vi "MCLScanAll.vi"() -> ()   [LabVIEW 2013]
uses:
  <vilib>/Analysis/NI_AALBase.lvlib
  <vilib>/Analysis/baseanly.llb/Mean (DBL).vi
  <vilib>/vision/NI_Vision_Development_Module.lvlib
  <vilib>/vision/Image Controls.llb/IMAQ Image.ctl
panel:
  in  "MCLScanning":bool
  in  "In Images":T2
  in  "APD 2 Cts":dbl[](array[numeric])
  in  "Trap Raw":waveform(dbl)[](array[waveform])
  in  "APD 1 Cts":dbl[](array[numeric])
  in  "Scan steps (MCL)":u64=40 caption="Scan steps (x)"
  in  "N APD Samp/step":dbl=3.0
  in  "Scan lines (y)":u64=20
  out "Cycles/step (MCL)":u64=2000 caption="Cycles/step" format="%.0p"
  out "Data map":dbl[][](graph)=[[-0.01671932143166878, -0.016392818706373227, -0.016060241502617766, -0.016885058281480972, -0.016633639866051188, -0.01614297111485056, -0.01624632439809061, -0.016223291898502697, -0.016322135358181895, -0.015998827366942206, -0.01674383457317074, -0.016349622303473588, -0.01611571290004051, -0.015972334649942688, -0.016306900004507047, -0.016265804263496074, -0.0160006281874421, -0.01579815848604542, -0.015557994770877373, -0.01623934207097493], [-0.016401746716030643, -0.016486228679580477, -0.016405819418185925, -0.017006941359896506, -0.01609698301441303, -0.0159938373980257, -0.015449969664593804, -0.016068061784641922, -0.016115383931390913, -0.015648222289449794, -0.01653040435156989, -0.01664368093936457, -0.015976629115606142, -0.015769041987412753, -0.015716784490458328, -0.016104708313091028, -0.015807740113897233, -0.016007795937736217, -0.015716865824611653, -0.016131560547170874], [-0.016881180243279052, -0.016682362901092443, -0.01653521208533211, -0.016569663649832547, -0.016584350108926265, -0.015788034358096, -0.01572997381191265, -0.016848256863673278, -0.016450971094654886, -0.016646544202256155, -0.016533647976865372, -0.01643411945121718, -0.01642968729491641, -0.015287525792493872, -0.015664412933211656, -0.016705160893495323, -0.01634751515697455, -0.016385950364931786, -0.01641611962972788, -0.016336369365154098], [-0.016944386833653874, -0.017209095062396696, -0.01643647162326984, -0.0169434622427136, -0.01645749558522405, -0.016283892481898044, -0.016603972603686925, -0.016019804038190342, -0.01633990863890397, -0.016779562572954584, -0.01649257003377154, -0.01633196294664365, -0.01681717360495772, -0.016151141680784836, -0.015631110690343758, -0.01616762209708058, -0.01570812545409377, -0.016238042109499973, -0.016140009377557954, -0.015480352129179791], [-0.016627380272623872, -0.016987040432100503, -0.0162998105424607, -0.01635693474229572, -0.016728613514399027, -0.015877063835195653, -0.01632422175035657, -0.015987062444069455, -0.016082210905250194, -0.016795453503208664, -0.0170165982501747, -0.016041147401410074, -0.015844635002206515, -0.01588368721722097, -0.016415515701510675, -0.01625686223052733, -0.015522307984761095, -0.016125254990784654, -0.016133227363549094, -0.016093654313254407], [-0.016918226627058684, -0.016546339201955095, -0.016238630263811032, -0.01698719582491472, -0.016111760237599002, -0.016169388046078873, -0.01635628471807927, -0.016477982760217016, -0.016022494806163096, -0.01635452184408291, -0.016437829589091835, -0.01620151587720066, -0.016192846971583803, -0.016361330735626047, -0.015920360440429684, -0.015596058601637491, -0.015839057608204695, -0.01590683226225114, -0.016147455226815495, -0.016061133185195295], [-0.016634948322751798, -0.016569012123295146, -0.01662465918442623, -0.01677966319575081, -0.016244237674368125, -0.016934028324529424, -0.015994902143504568, -0.01577806108898649, -0.015702882269567658, -0.01637426003303808, -0.016516796952512437, -0.01646180977161214, -0.017050841082784957, -0.015210920961454804, -0.016180578875882937, -0.01607665952058283, -0.01643056573904152, -0.01624726697921726, -0.016811320756287537, -0.015704237088347145], [-0.016797771368752906, -0.01616083928333069, -0.016453251971550422, -0.01638112181272177, -0.01590261356594244, -0.01608147749759244, -0.016020370516697566, -0.01666407664114518, -0.01638481284701757, -0.016175328500489604, -0.015634096607040564, -0.01659680945708638, -0.01626086024191585, -0.016096523812787963, -0.015760521307245458, -0.01615157630765101, -0.01563169067138887, -0.016252628883934674, -0.016238504839935688, -0.016296984466382107], [-0.01667963634531472, -0.015869270181190567, -0.01639782773103042, -0.01636439382881424, -0.01666285543553242, -0.016692875783958446, -0.016121724588237546, -0.016079967645743654, -0.01632967716613466, -0.0165840590606689, -0.01625421166976198, -0.016098422085292646, -0.016839026057991122, -0.01618499247497865, -0.015391600029151147, -0.016339655626827314, -0.015612166346566772, -0.015935379715422582, -0.015751812989013417, -0.016043659821299468], [-0.016548348623009697, -0.016991017407413864, -0.016507403110123067, -0.016536793878207376, -0.016691120016137963, -0.01577327808799238, -0.016241167864690632, -0.016068735698142586, -0.015840387814149363, -0.016134357225980472, -0.015841333026290365, -0.0163038114660657, -0.01664004009343323, -0.015517995684912076, -0.01510255011893393, -0.016011490555515644, -0.01579492187645071, -0.016061693314939115, -0.016070791499276448, -0.015958266458419586], [-0.017158052821315092, -0.016990745992594425, -0.01659770916824297, -0.016038631482428484, -0.016146804022232154, -0.01576224906436341, -0.016188682344964726, -0.016682643876198163, -0.016363274145684666, -0.01639850086318443, -0.015896821220835786, -0.015725853678146523, -0.01601090474694708, -0.015561700057052, -0.015999978841264924, -0.01601836056022779, -0.016765653382201824, -0.016096916088969352, -0.016073837821775124, -0.015692878955540758], [-0.01663419671959083, -0.016709422884628247, -0.017440867448447667, -0.016794212435564802, -0.016747490720603195, -0.017381751349696366, -0.016447004176656708, -0.016200072448833015, -0.016045160782039845, -0.01632124390318996, -0.01679169430451878, -0.016160654157203025, -0.016749084172300182, -0.015317451826774697, -0.01616958983467165, -0.015522373654827837, -0.016042029406509332, -0.016273918604509642, -0.016417636335760946, -0.01644358854973573], [-0.016334373306253872, -0.016757773312361682, -0.016379901767213538, -0.016648254461466998, -0.016415141976627915, -0.016163802224577726, -0.01585938187523836, -0.01585373106879133, -0.015975877635193418, -0.01599748687305492, -0.016737850820893803, -0.01594503246026053, -0.01605934628998727, -0.0158171814426758, -0.015143820145612868, -0.016535815039113604, -0.01611350163485256, -0.01603586147994221, -0.016191023597649318, -0.015673182413705102], [-0.016700857633048308, -0.017051706885756718, -0.016395162126784154, -0.016864165985049667, -0.01667278712452, -0.016023236569300325, -0.015936447644162688, -0.01626053315184134, -0.016666644977778797, -0.01651990276982608, -0.01690611112853018, -0.016570014742366936, -0.016014494913507715, -0.016334286074074115, -0.01621235686701924, -0.01653022812336152, -0.01583634924223019, -0.016281303974484927, -0.01653990312391212, -0.015384206653677268], [-0.016471441301573585, -0.01647096314202187, -0.016715886966535524, -0.015878302888681167, -0.016818970876684446, -0.016713152489800882, -0.0154648252478201, -0.016328530500277577, -0.015836781582585016, -0.01591923201699931, -0.016315094505816256, -0.015951841421804724, -0.01608430179945204, -0.015957272458344565, -0.015751249520465478, -0.016350306857141315, -0.015517909552404317, -0.015884662571158274, -0.016211720964471307, -0.01537858018482844], [-0.01674440523726064, -0.016870567772511377, -0.016213148874409115, -0.016888734754126403, -0.017090609693170035, -0.01659256562080198, -0.01625635717081822, -0.016107107745803876, -0.016234190134722645, -0.016577197956586683, -0.01658670958631228, -0.016563728816596346, -0.016688515093891267, -0.016736196160361996, -0.015994597797780702, -0.016061666241292242, -0.015206770358209283, -0.01656914278587982, -0.01606315534154764, -0.015681866815853374], [-0.016944331036564515, -0.017205260427342613, -0.01677120483170293, -0.016402843466637763, -0.01674116281665193, -0.016423395631415146, -0.01525500299962603, -0.01627542397053335, -0.016664853908603776, -0.01620332976021642, -0.015950564835878013, -0.01610107356411497, -0.016396683154864377, -0.015976631236977498, -0.015478300298060717, -0.015835627632208554, -0.01604600189786053, -0.015850180758366084, -0.01603596051783181, -0.015769623989901102], [-0.016857923835780924, -0.016573198672727902, -0.016660307411618773, -0.016198760579099178, -0.016151481374992453, -0.01623511193332007, -0.015818969815924802, -0.01644510963983431, -0.015972042272190907, -0.01666642359581892, -0.01666443700190194, -0.016438254918363447, -0.016138118663893655, -0.015691974269895034, -0.016587077315345165, -0.015965118060360686, -0.015699839910512218, -0.01561194620613338, -0.016186792034230305, -0.016197922335520733], [-0.016756662992071368, -0.017021980605505502, -0.01671540550240299, -0.016161860765568574, -0.016256637402529132, -0.01604906368842445, -0.016092507257301394, -0.01617438393323743, -0.016105543848009572, -0.016246592326198385, -0.016142744624025374, -0.016159689527728567, -0.016177575339496836, -0.015961391152738445, -0.015789242903564853, -0.016290502978789936, -0.01590902706214275, -0.016035878036151207, -0.0163699057102928, -0.016166856731619543], [-0.016230743921604517, -0.01699457586491366, -0.01691575006710251, -0.01691567874763252, -0.016632348348462205, -0.01564006866069024, -0.015669555325846102, -0.01675726036853814, -0.015659388136628594, -0.01633203630678029, -0.016275904140963263, -0.01599466989252362, -0.01670183436780044, -0.016544315654085533, -0.015882735536646285, -0.01634814491721433, -0.015693511174422668, -0.015857069610244905, -0.015293298228102974, -0.01570879180052374], [-0.016746550537387085, -0.016635756849929545, -0.01704192789682773, -0.01592942336549498, -0.016565335498658518, -0.016559981627150607, -0.016370390094235444, -0.016204117687222342, -0.01636993721064581, -0.016019023809705737, -0.01624713908528634, -0.01653713290533686, -0.01654191191022731, -0.015871787270804183, -0.016600435605206076, -0.016053794928515903, -0.015786397557799592, -0.016167422435048453, -0.016149009764007245, -0.015779827376486453], [-0.017141787830569893, -0.01685604196926299, -0.016770676218784503, -0.01657265724540346, -0.016973351148096293, -0.016347677914333066, -0.015700463473615457, -0.0157292679709582, -0.016282549721629708, -0.015799962485816943, -0.0169651499113691, -0.017005390716294616, -0.01616841590634147, -0.01579805772887789, -0.015884669429112312, -0.01687947774540062, -0.015546104827296667, -0.01606408203496036, -0.015764690031214893, -0.016077969368821936], [-0.01755128513645066, -0.016614441354853425, -0.01642295621649906, -0.016572002735089818, -0.016539344978417192, -0.01665672671509038, -0.01610564101766388, -0.0167710479608722, -0.01604147346071364, -0.015915051759660022, -0.01690954942974296, -0.01618215110656205, -0.01687103577661275, -0.015704550539293104, -0.01567934362211993, -0.015968805810754147, -0.01586985536309292, -0.015848872001954256, -0.015923479964089694, -0.015604572794266433], [-0.01700702905775247, -0.016405242404623068, -0.016957584669743626, -0.01649808356316003, -0.015831866505709048, -0.01650461850371917, -0.015987113078007254, -0.015834023912635466, -0.015505062044615166, -0.016233666617861173, -0.016028249584376462, -0.016292798595496677, -0.016811560188299345, -0.015802581883183398, -0.015195148613460024, -0.015765465657774175, -0.016294889918615045, -0.01647530657977607, -0.016354233471026363, -0.01618598563271133], [-0.016283357847285636, -0.01655641981831666, -0.016127059444156554, -0.016293855360523378, -0.01631947219897442, -0.016398508430939616, -0.0164960599809452, -0.01635229032278839, -0.016150072161158744, -0.01646190473964058, -0.016283962555137702, -0.01689040784367708, -0.016767163139998632, -0.016438000493173108, -0.015954956500429416, -0.016569056147695202, -0.016605504963760735, -0.015329313107534112, -0.01578842030659742, -0.015421959499234628], [-0.016479987599589248, -0.01644678482494596, -0.016512996052180717, -0.01623094473834884, -0.016604746810030113, -0.016230213519226107, -0.016359208382350467, -0.01609761921903255, -0.016464485575532387, -0.015985272322973462, -0.015774520381458212, -0.01632178510310122, -0.016823351362691343, -0.01643553466150876, -0.015434648968053383, -0.01640702032901096, -0.015639626970513753, -0.01608966370811705, -0.016018362361111357, -0.01607982188546427], [-0.016959739645157706, -0.016680901866661726, -0.015836205448559966, -0.016650560318028734, -0.015979362423611275, -0.015641297610719303, -0.015788746501915876, -0.016033508703118756, -0.01595573902096323, -0.016363948579213562, -0.016349864006002027, -0.016495398899173445, -0.016242648234899834, -0.016920033344786076, -0.016276181128461735, -0.016473741446416813, -0.015963577017676644, -0.015565621002678179, -0.01634988477510272, -0.016759987490697584], [-0.016465195958807775, -0.016666490625723715, -0.016658908615375, -0.01597417902764041, -0.016394946754303752, -0.016153528909152313, -0.016275277887248356, -0.016575820504070977, -0.016165440248126276, -0.0158334592734765, -0.016393067206609387, -0.016885479811953534, -0.016471593134372298, -0.017124297138208497, -0.01548599428740715, -0.016309544928836586, -0.015739577267293366, -0.016315386973421362, -0.016361118135948566, -0.016635949477566882], [-0.016680470580762462, -0.016967020008211, -0.017070403001069857, -0.015793158201855152, -0.01661718510493328, -0.01621301409151063, -0.015497330917384148, -0.016267684516616924, -0.015545683307124036, -0.01584462817622427, -0.016830529260392843, -0.016203294725707643, -0.016943290418910587, -0.015581438668509352, -0.015578492450734066, -0.01643368853494311, -0.016285119780950222, -0.015912568651561352, -0.015719368411857025, -0.015732642681635923], [-0.017056323385982973, -0.017071971641855074, -0.01624203196673346, -0.016577086084052214, -0.016198385464505236, -0.015959998936922397, -0.015388246890736087, -0.01690871560472578, -0.016520770777269024, -0.016719342780151844, -0.01589885976225658, -0.016316317143634285, -0.015927259253864068, -0.01613903479860508, -0.015938319643326725, -0.015996730877187566, -0.01552190097834432, -0.016279927776335308, -0.015995176436170485, -0.015804091652970826], [-0.017190435316337342, -0.016575163169333516, -0.01629659819256952, -0.016774256975583077, -0.015978440181354282, -0.016162892801179076, -0.01620143768882657, -0.016215940324925678, -0.016085616640623322, -0.01624795446292185, -0.015590279490139558, -0.016351775677783426, -0.01628162630120476, -0.016736583715483217, -0.015290607493835316, -0.01675006130238602, -0.016112399997689694, -0.016085396155956493, -0.01584495781031281, -0.016031709625742012], [-0.017226310157841672, -0.0164663033859778, -0.01638852606295136, -0.01642215259901681, -0.016566243818266997, -0.016484045986143257, -0.016452209817223822, -0.016464707609223313, -0.01598467645947642, -0.016476401570535384, -0.015529223129381136, -0.016802343788985992, -0.016417294815804, -0.016305476633183012, -0.015407470515554668, -0.01588918182788552, -0.015839354895906106, -0.016859219988342257, -0.016188952756112908, -0.015382351679335257], [-0.017044276140355946, -0.016525294382434108, -0.01600036800318285, -0.01692841042125611, -0.016063543400203904, -0.0167008216867912, -0.01583944304325613, -0.015982843969462788, -0.01610446772754332, -0.01650934416727942, -0.016660683575282727, -0.016326108469991264, -0.01614299940648814, -0.016050548764700443, -0.016131072933532012, -0.016315196635999143, -0.016225473554238007, -0.01551847935196565, -0.015874550726858914, -0.01566897000262655], [-0.016174756903461544, -0.01692999553661901, -0.01705167048362926, -0.01660949009366751, -0.016107419352032235, -0.016188509519945497, -0.015585853922651487, -0.01612262091090234, -0.016426426055949322, -0.01609822137272688, -0.016735004284984756, -0.016043599908818165, -0.016651804571551146, -0.01556136051538674, -0.015408827232157843, -0.015855874683892428, -0.015887023972496795, -0.01599811437353065, -0.015655637769778918, -0.015893480415302176], [-0.016396467105890343, -0.01690556505247584, -0.0163054855200399, -0.016446662941364928, -0.01622691165873451, -0.016690239637868323, -0.015785441074554568, -0.016620593981308673, -0.015765446409343138, -0.016270811628848948, -0.016094841434208293, -0.01632812303243944, -0.01619217328151394, -0.015836234359203484, -0.016074598803568225, -0.01532030760600064, -0.01657169575010852, -0.016393493124135967, -0.01597552762388542, -0.015565046037824628], [-0.016299520764774443, -0.016637551393085426, -0.016299287907039765, -0.01610813956937386, -0.016305200311999217, -0.016601228593523636, -0.016288899767132464, -0.016305235511310533, -0.016063090550620947, -0.01683118193989227, -0.015518909238992087, -0.01620458965118359, -0.01645647074542291, -0.015677575909554008, -0.015332584749786342, -0.016079840062543812, -0.016278322310175185, -0.01605786016548567, -0.01657700147769983, -0.01606751816440997], [-0.016441387384698882, -0.017325914631361444, -0.017225293509456174, -0.016118796157285526, -0.016362377734664042, -0.01516634537172325, -0.01608508664570788, -0.01572299536201756, -0.01616493137153105, -0.01621315960010322, -0.016750280429064943, -0.016228195768808316, -0.01653543568323192, -0.01645026349483051, -0.016050647149129828, -0.01642593239180811, -0.0161192309302286, -0.01629438826737352, -0.015557310160813994, -0.016021567325025916], [-0.01686693458295582, -0.016740786564424494, -0.01648453245605215, -0.01640092243822592, -0.01555424864442638, -0.01667099748425638, -0.016069415470156286, -0.01638225749592203, -0.01607630099787768, -0.01614344420814296, -0.016216929728619375, -0.016309670684273796, -0.015741358140653132, -0.015770999475234804, -0.01601963602183988, -0.01615265943136728, -0.016152653946118384, -0.01698528285009184, -0.015969420465915152, -0.01578449323306024], [-0.01598619419452168, -0.016362732490235912, -0.016433844312774552, -0.016357999277320685, -0.015969441982301692, -0.01621147526376268, -0.016085473373391473, -0.016306341052304336, -0.015855664982231947, -0.015900633884010838, -0.016902356755211914, -0.016434765274207237, -0.016180164153866673, -0.015973977144992546, -0.01589274164800459, -0.01640268056199417, -0.016415161422386984, -0.01617112040367598, -0.016354725082739732, -0.016206639631885546], [-0.016048964224847716, -0.016745007333129024, -0.017180534108641177, -0.016329775174222558, -0.016582289070660373, -0.016075138720435006, -0.016345162602564738, -0.016090296577092385, -0.016153752753705675, -0.016379459268123033, -0.016228628993078524, -0.016712275509199688, -0.015795168051192618, -0.015386431874568587, -0.01610093851445945, -0.01633598707495066, -0.015921284689633122, -0.016330315102764423, -0.015994974665173196, -0.015537812293197398]]
  out "Waveform Graph":dbl[](graph)=[5.0, 4.0, 2.0, 2.0, 5.0, 3.0, 2.0, 4.0, 0.0, 5.0, 4.0, 3.0, 5.0, 2.0, 4.0, 1.0, 5.0, 3.0, 0.0, 2.0, 2.0, 4.0, 2.0, 1.0, 2.0, 8.0, 2.0, 4.0, 4.0, 3.0, 3.0, 1.0, 5.0, 5.0, 3.0, 2.0, 7.0, 2.0, 4.0, 4.0, 1.0, 1.0, 3.0, 4.0, 3.0, 9.0, 0.0, 6.0, 4.0, 5.0, 2.0, 4.0, 4.0, 4.0, 4.0, 2.0, 3.0, 6.0, 3.0, 4.0, 4.0, 5.0, 5.0, 8.0, 5.0, 4.0, 4.0, 7.0, 4.0, 3.0, 1.0, 4.0, 5.0, 4.0, 2.0, 3.0, 3.0, 1.0, 2.0, 1.0] caption="APD Line Scan"
  in  "Channel":i32=4
  out "Detection Laser X":T1(plugin-control)
  out "APD 1":T1(plugin-control) caption="APD 1 (Cy3)"
  out "Detection Laser Y":T1(plugin-control)
  out "APD 2":T1(plugin-control) caption="APD 2 (Cy5)"
types:
  T1 = typedef "IMAQ Image.ctl" = refnum<image>
  T2 = cluster{"New Image":T1, "New Image":T1, "New Image":T1, "New Image":T1}
  T3 = cluster{"Origin Pixel":cluster{"X":sgl, "Y":sgl}, "Angle Relative to Horizontal (deg)":sgl, "Axis Reference":u32}
  T4 = typedef "Simple Grid Descriptor" = cluster{"X Step":sgl, "Y Step":sgl, "Unit":T5}
  T5 = typedef "Image Unit" = enum32{"Undefined", "Angström", "Micrometer", "Millimeter", "Centimeter", "Meter", "Kilometer", "Microinch", "Inch", "Feet", "Nautical miles", "Standard miles", "Steps"}
diagram:
  w18 = u32 0 items=["Horizontal", "Vertical", "Central", "1st Diagonal", "2nd Diagonal"] ("Type of Symmetry")
  w44 = u32 0 items=["Horizontal", "Vertical", "Central", "1st Diagonal", "2nd Diagonal"] ("Type of Symmetry")
  w47 = u32 0 items=["Horizontal", "Vertical", "Central", "1st Diagonal", "2nd Diagonal"] ("Type of Symmetry")
  w76 = u32 0 items=["Horizontal", "Vertical", "Central", "1st Diagonal", "2nd Diagonal"] ("Type of Symmetry")
  n1 = local read "Scan lines (y)"() -> (w7:u64)
  n2 = local read "Cycles/step (MCL)"() -> (w61:u64)
  n3 = Index Array(array="Trap Raw", index=10) -> (element=w110:waveform(dbl))
  n4 = Index Array(array="Trap Raw", index=11) -> (element=w107:waveform(dbl))
  n5 = Index Array(array="Trap Raw", index="Channel") -> (element=w106:waveform(dbl))
  n6 = Unbundle("In Images") -> ("New Image"=w11:T1, "New Image"=w10:T1, "New Image"=w9:T1, "New Image"=w8:T1)
  n7 = Unbundle By Name(w110) -> ("Y"=w63:dbl[])
  n8 = Unbundle By Name(w107) -> ("Y"=w65:dbl[])
  n9 = Unbundle By Name(w106) -> ("Y"=w70:dbl[])
  n10 = call "downsample 1D array - double.vi"("Ave N"=w61, "Array In"=w63) -> ("Array Out"=w62:dbl[])  [unwired: 1 out]
  n11 = call "downsample 1D array - double.vi"("Ave N"=w61, "Array In"=w65) -> ("Array Out"=w64:dbl[])  [unwired: 1 out]
  n12 = call "downsample 1D array - double.vi"("Ave N"=w61, "Array In"=w70) -> ("Array Out"=w69:dbl[])  [unwired: 1 out]
  n13 = local read "Scan steps (MCL)"() -> (w20:u64)
  n14 = local read "N APD Samp/step"() -> (w22:dbl)
  n15 = feedback #1("APD 1 Cts") -> (w130:dbl[])
  n16 = Build Array (concatenate)(w130, "APD 1 Cts") -> (w112:dbl[])
  n17 = feedback #2("APD 2 Cts") -> (w38:dbl[])
  n18 = Build Array (concatenate)(w38, "APD 2 Cts") -> (w37:dbl[])
  n19 = Select(t="APD 1 Cts", s="MCLScanning", f=w112) -> (s? t:f=w116:dbl[])
  n20 = feedback-in #1(w116) -> ()
  n21 = Select(t="APD 2 Cts", s="MCLScanning", f=w37) -> (s? t:f=w21:dbl[])
  n22 = feedback-in #2(w21) -> ()
  n23 = feedback #3(w62) -> (w118:dbl[])
  n24 = Build Array (concatenate)(w118, w62) -> (w109:dbl[])
  n25 = feedback #4(w69) -> (w128:dbl[])
  n26 = Build Array (concatenate)(w128, w69) -> (w127:dbl[])
  n27 = feedback #5(w64) -> (w120:dbl[])
  n28 = Build Array (concatenate)(w120, w64) -> (w121:dbl[])
  n29 = Select(t=w64, s="MCLScanning", f=w121) -> (s? t:f=w67:dbl[])
  n30 = feedback-in #5(w67) -> ()
  n31 = Select(t=w62, s="MCLScanning", f=w109) -> (s? t:f=w66:dbl[])
  n32 = feedback-in #3(w66) -> ()
  n33 = Select(t=w69, s="MCLScanning", f=w127) -> (s? t:f=w68:dbl[])
  n34 = feedback-in #4(w68) -> ()
  n35 = Multiply(x=w20, y=u64 2) -> (x*y=w6:u64)
  n36 = call "integrate 1D array interval - double.vi"("Ave N"=w22, "Array In"=w21) -> ("Array Out"=w33:dbl[])  [unwired: 1 out]
  n37 = call "integrate 1D array interval - double.vi"("Ave N"=w22, "Array In"=w116) -> ("Array Out"=w115:dbl[])  [unwired: 1 out]
  n38 = Array Size(array=w33) -> (size(s)=w34:i32)
  n39 = Array Size(array=w115) -> (size(s)=w117:i32)
  n40 = Multiply(x=w7, y=w6) -> (x*y=w36:u64)
  n41 = Multiply(x=w7, y=w6) -> (x*y=w125:u64)
  n42 = call-poly <vilib>:"Mean.vi"("X"=w66) -> ("mean"=w50:dbl)  [unwired: 1 out]
  n43 = Subtract(x=w36, y=w34) -> (x-y=w27:u64)
  n44 = call-poly <vilib>:"Mean.vi"("X"=w68) -> ("mean"=w55:dbl)  [unwired: 1 out]
  n45 = call-poly <vilib>:"Mean.vi"("X"=w67) -> ("mean"=w53:dbl)  [unwired: 1 out]
  n46 = call-poly <vilib>:"Mean.vi"("X"=w33) -> ("mean"=w24:dbl)  [unwired: 1 out]
  n47 = Subtract(x=w125, y=w117) -> (x-y=w60:u64)
  n48 = call-poly <vilib>:"Mean.vi"("X"=w115) -> ("mean"=w57:dbl)  [unwired: 1 out]
  n49 = Initialize Array(1.0 ("element"), w27) -> (w23:dbl[])
  n50 = Initialize Array(1.0 ("element"), w60) -> (w51:dbl[])
  n51 = Multiply(x=w23, y=w24) -> (x*y=w25:dbl[])
  n52 = Multiply(x=w51, y=w53) -> (x*y=w54:dbl[])
  n53 = Multiply(x=w51, y=w55) -> (x*y=w56:dbl[])
  n54 = Multiply(x=w51, y=w50) -> (x*y=w52:dbl[])
  n55 = Multiply(x=w51, y=w57) -> (x*y=w58:dbl[])
  n56 = Build Array (concatenate)(w66, w52) -> (w119:dbl[])
  n57 = Build Array (concatenate)(w68, w56) -> (w123:dbl[])
  n58 = Build Array (concatenate)(w67, w54) -> (w122:dbl[])
  n59 = Build Array (concatenate)(w33, w25) -> (w35:dbl[])
  n60 = Build Array (concatenate)(w115, w58) -> (w124:dbl[])
  n61 = Reshape Array(w119, w7, w6) -> (w86:dbl[][])
  n62 = Reshape Array(w35, w7, w6) -> (w31:dbl[][])
  n63 = Reshape Array(w123, w7, w6) -> (w78:dbl[][])
  n64 = Reshape Array(w122, w7, w6) -> (w93:dbl[][])
  n65 = Reshape Array(w124, w7, w6) -> (w103:dbl[][])
  n66 = Array Subset(array=w93, index (col)=0 ("index"), length (col)=w20) -> (w98:dbl[][])  [unwired: 2 in]
  n67 = Array Subset(array=w93, index (col)=w20) -> (w96:dbl[][])  [unwired: 3 in]
  n68 = Array Subset(array=w78, index (col)=0 ("index"), length (col)=w20) -> (w84:dbl[][])  [unwired: 2 in]
  n69 = Array Subset(array=w78, index (col)=w20) -> (w82:dbl[][])  [unwired: 3 in]
  n70 = Array Subset(array=w31, index (col)=0 ("index"), length (col)=w20) -> (w30:dbl[][])  [unwired: 2 in]
  n71 = Array Subset(array=w31, index (col)=w20) -> (w28:dbl[][])  [unwired: 3 in]
  n72 = Array Subset(array=w103, index (col)=0 ("index"), length (col)=w20) -> (w102:dbl[][])  [unwired: 2 in]
  n73 = Array Subset(array=w103, index (col)=w20) -> (w100:dbl[][])  [unwired: 3 in]
  n74 = Array Subset(array=w86, index (col)=0 ("index"), length (col)=w20) -> (w91:dbl[][])  [unwired: 2 in]
  n75 = Array Subset(array=w86, index (col)=w20) -> (w89:dbl[][])  [unwired: 3 in]
  n76 = for {
    tunnel: w98 -> [w132] mode=indexing
    tunnel: [w131] -> w97 mode=indexing
    workers-P: _ -> [_]
    n77 = Reverse 1D Array(array=w132) -> (reversed array=w131:dbl[])
  }
  n78 = for {
    tunnel: w84 -> [w134] mode=indexing
    tunnel: [w133] -> w83 mode=indexing
    workers-P: _ -> [_]
    n79 = Reverse 1D Array(array=w134) -> (reversed array=w133:dbl[])
  }
  n80 = for {
    tunnel: w30 -> [w136] mode=indexing
    tunnel: [w135] -> w29 mode=indexing
    workers-P: _ -> [_]
    n81 = Reverse 1D Array(array=w136) -> (reversed array=w135:dbl[])
  }
  n82 = for {
    tunnel: w102 -> [w138] mode=indexing
    tunnel: [w137] -> w101 mode=indexing
    workers-P: _ -> [_]
    n83 = Reverse 1D Array(array=w138) -> (reversed array=w137:dbl[])
  }
  n84 = for {
    tunnel: w91 -> [w140] mode=indexing
    tunnel: [w139] -> w90 mode=indexing
    workers-P: _ -> [_]
    n85 = Reverse 1D Array(array=w140) -> (reversed array=w139:dbl[])
  }
  n86 = Index Array(array=w103, index (row)=0) -> (element=→"Waveform Graph":dbl[])  [unwired: 1 in]
  n87 = Add(x=w97, y=w96) -> (x+y=w95:dbl[][])
  n88 = Add(x=w83, y=w82) -> (x+y=w81:dbl[][])
  n89 = Add(x=w29, y=w28) -> (x+y=w13:dbl[][])
  n90 = Add(x=w101, y=w100) -> (x+y=w75:dbl[][])
  n91 = Add(x=w90, y=w89) -> (x+y=w88:dbl[][])
  n92 = Divide(x=w81, y=2) -> (x/y=w79:dbl[][])
  n93 = Divide(x=w95, y=2) -> (x/y=w40:dbl[][])
  n94 = Divide(x=w88, y=2) -> (x/y=w42:dbl[][])
  n95 = To Single Precision Float(number=w75) -> (single precision float=w74:sgl[][])
  n96 = Transpose 2D Array(2D array=w79) -> (transposed array=→"Data map":dbl[][])
  n97 = To Single Precision Float(number=w13) -> (single precision float=w17:sgl[][])
  n98 = To Single Precision Float(number=w40) -> (single precision float=w46:sgl[][])
  n99 = To Single Precision Float(number=w42) -> (single precision float=w43:sgl[][])
  n100 = call "IMAQ ArrayToImage"("Image Pixels (Float)"=w74, "Image"=w11) -> ("Image Out"=w77:T1)  [unwired: 8 in, 1 out]
  n101 = call "IMAQ ArrayToImage"("Image Pixels (Float)"=w17, "Image"=w10) -> ("Image Out"=w19:T1)  [unwired: 8 in, 1 out]
  n102 = call "IMAQ ArrayToImage"("Image Pixels (Float)"=w46, "Image"=w9) -> ("Image Out"=w48:T1)  [unwired: 8 in, 1 out]
  n103 = call "IMAQ ArrayToImage"("Image Pixels (Float)"=w43, "Image"=w8) -> ("Image Out"=w45:T1)  [unwired: 8 in, 1 out]
  n104 = call "IMAQ Symmetry"("Type of Symmetry"=w76, "Image Src"=w77) -> ("Image Dst Out"=w72:T1)  [unwired: 3 in, 1 out]
  n105 = call "IMAQ Symmetry"("Type of Symmetry"=w18, "Image Src"=w19) -> ("Image Dst Out"=w15:T1)  [unwired: 3 in, 1 out]
  n106 = call "IMAQ Symmetry"("Type of Symmetry"=w47, "Image Src"=w48) -> ("Image Dst Out"=→"Detection Laser X":T1)  [unwired: 3 in, 1 out]
  n107 = call "IMAQ Symmetry"("Type of Symmetry"=w44, "Image Src"=w45) -> ("Image Dst Out"=→"Detection Laser Y":T1)  [unwired: 3 in, 1 out]
  n108 = call "IMAQ Set Simple Calibration"("Calibration Axis Info"=T3 {"Origin Pixel"={"X"=0.0, "Y"=0.0}, "Angle Relative to Horizontal (deg)"=0.0, "Axis Reference"=0}, "Grid Descriptor"=T4 {"X Step"=0.3, "Y Step"=0.3, "Unit"=enum."Undefined"}, "Image"=w72) -> ("Calibrated Image"=→"APD 1":T1)  [unwired: 7 in, 1 out]
  n109 = call "IMAQ Set Simple Calibration"("Calibration Axis Info"=T3 {"Origin Pixel"={"X"=0.0, "Y"=0.0}, "Angle Relative to Horizontal (deg)"=0.0, "Axis Reference"=0}, "Grid Descriptor"=T4 {"X Step"=0.3, "Y Step"=0.3, "Unit"=enum."Undefined"}, "Image"=w15) -> ("Calibrated Image"=→"APD 2":T1)  [unwired: 7 in, 1 out]
